vi "Initialize-message-queues.vi"(8 "error in":errorcluster, 9 "Queue depth (15)":i32=15, 11 "Data ref. in":refnum<data-value>) -> (0 "error IO":errorcluster, 2 "Queue out":refnum<queue>, 3 "Data ref.":refnum<data-value>)   [LabVIEW 2013, in "CameraVision.lvlib" / "CV-Main.lvclass"]
uses:
  CV-Main.lvclass
  Main-actions.ctl
  CV-Main.lvclass/CV-Main.ctl
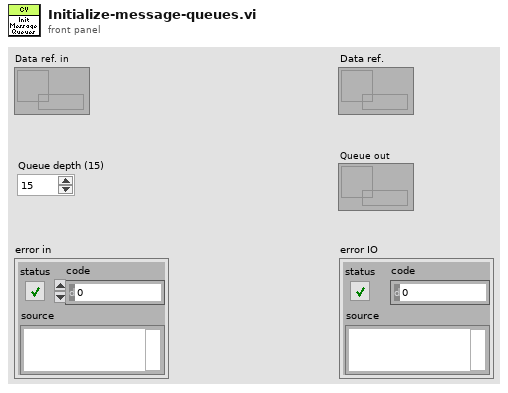
[diagram p1: front panel]
types:
  T1 = typedef "CameraVision.lvlib/CV-Main.lvclass/Main-actions.ctl" = enum16{"Idle", "Initialize", "Load defaults", "Update settings", "Check settings", "Save settings", "Save settings with dialog", "Load settings", "Load data", "Activate", "Start", "Wait for start signal", "Acquire & process", "Iterate", "Stop", "Refresh display", "Refresh status", "View camera settings", "View grabber settings", "Exit"}
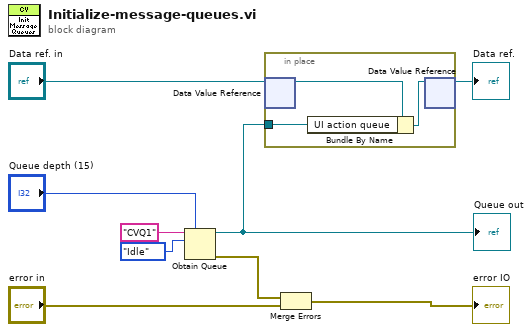
[diagram p0: block diagram]
diagram:
  n1 = Obtain Queue(max queue size (-1, unlimited)="Queue depth (15)", name (unnamed)="CVQ1", element data type=Main-actions."Idle" ("MainStateSelector")) -> (queue out=w1:refnum<queue>, error out=w9:errorcluster)  [unwired: 2 in, 1 out]
  "Queue out" <- w1
  n2 = in-place {
    in-place-border: w1 -> [w10]
    n3 = in-place-dvr #1("Data ref. in") -> (w12:refnum<class "CV-Main.lvclass">)  [unwired: 1 out]
    n4 = Bundle By Name(cluster=w12, "UI action queue"=w10) -> (w11:refnum<class "CV-Main.lvclass">)
    n5 = in-place-dvr #1(w11) -> (→"Data ref.":refnum<data-value>)  [unwired: 1 out]
  }
  n6 = Merge Errors(w9, "error in") -> (→"error IO":errorcluster)
